vi "Attitude_ODE.vi"() -> ()   [LabVIEW 2018]
uses:
  <vilib>/Analysis/coordinate.llb/Euler Rotation Order.ctl
  <vilib>/imath/engines/lvmath2/RunTimeEngine/IndexRead/NIMS M(S,S).vi
  <instcachedir>/0/NIMS M(S,S)_AC51E74150A542F7991B9634C66F3096.lvgen/NIMS M(S,S)_AC51E74150A542F7991B9634C66F3096_002.vi
  <vilib>/imathl/engines/lvmath/Functions/Error Handling/Create Error.vi
  <vilib>/imath/engines/lvmath2/RunTimeEngine/IndexRead/NIMS V(S).vi
  <instcachedir>/0/NIMS V(S)_0488751826AF41519A22953C041130DC.lvgen/NIMS V(S)_0488751826AF41519A22953C041130DC_002.vi
  <vilib>/imath/engines/lvmath2/RunTimeEngine/ErrorHandling/NIMS_Create Error From Enums.vi
  <vilib>/imath/engines/lvmath2/RunTimeEngine/ArithmeticOperatorToken/NIMS_ArithmeticOperator_multmx-internal.vi
  <instcachedir>/0/NIMS_ArithmeticOperator_multmx-internal_16A6E1DA326644AB974D30232E729C42.lvgen/NIMS_ArithmeticOperator_multmx-internal_16A6E1DA326644AB974D30232E729C42_011.vi
  <instcachedir>/0/NIMS M(S,S)_AC51E74150A542F7991B9634C66F3096.lvgen/NIMS M(S,S)_AC51E74150A542F7991B9634C66F3096_000.vi
  <vilib>/imath/engines/lvmath2/RunTimeEngine/NodeEndStatement/NIMS_NodeEndStatement_Output.vi
  <instcachedir>/0/NIMS_NodeEndStatement_Output_53EC0D466D134D7ABD903AC30B43404B.lvgen/NIMS_NodeEndStatement_Output_53EC0D466D134D7ABD903AC30B43404B_005.vi
  <instcachedir>/0/NIMS_NodeEndStatement_Output_53EC0D466D134D7ABD903AC30B43404B.lvgen/NIMS_NodeEndStatement_Output_53EC0D466D134D7ABD903AC30B43404B_011.vi
  <vilib>/imath/engines/lvmath2/RunTimeEngine/ErrorHandling/NIMS_Finalize Error.vi
  <instcachedir>/0/NIMS_NodeEndStatement_Output_53EC0D466D134D7ABD903AC30B43404B.lvgen/NIMS_NodeEndStatement_Output_53EC0D466D134D7ABD903AC30B43404B_002.vi
  <vilib>/gmath/NI_Gmath.lvlib
  <vilib>/Analysis/NI_AALPro.lvlib
panel:
  out "Euler Angles":cluster{"phi":dbl, "theta":dbl, "psi":dbl}
  in  "stop":bool
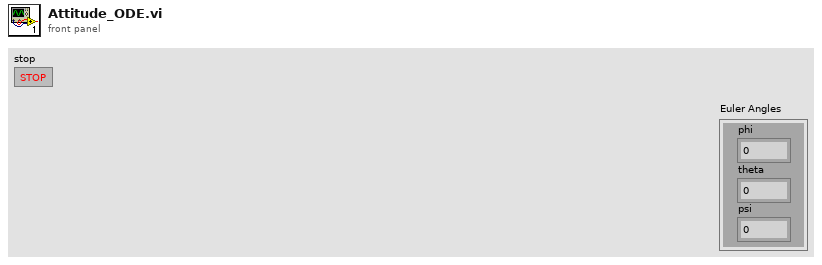
[diagram p1: front panel]
types:
  T1 = typedef "NI_AALPro.lvlib/Euler Rotation Order.ctl" = u16
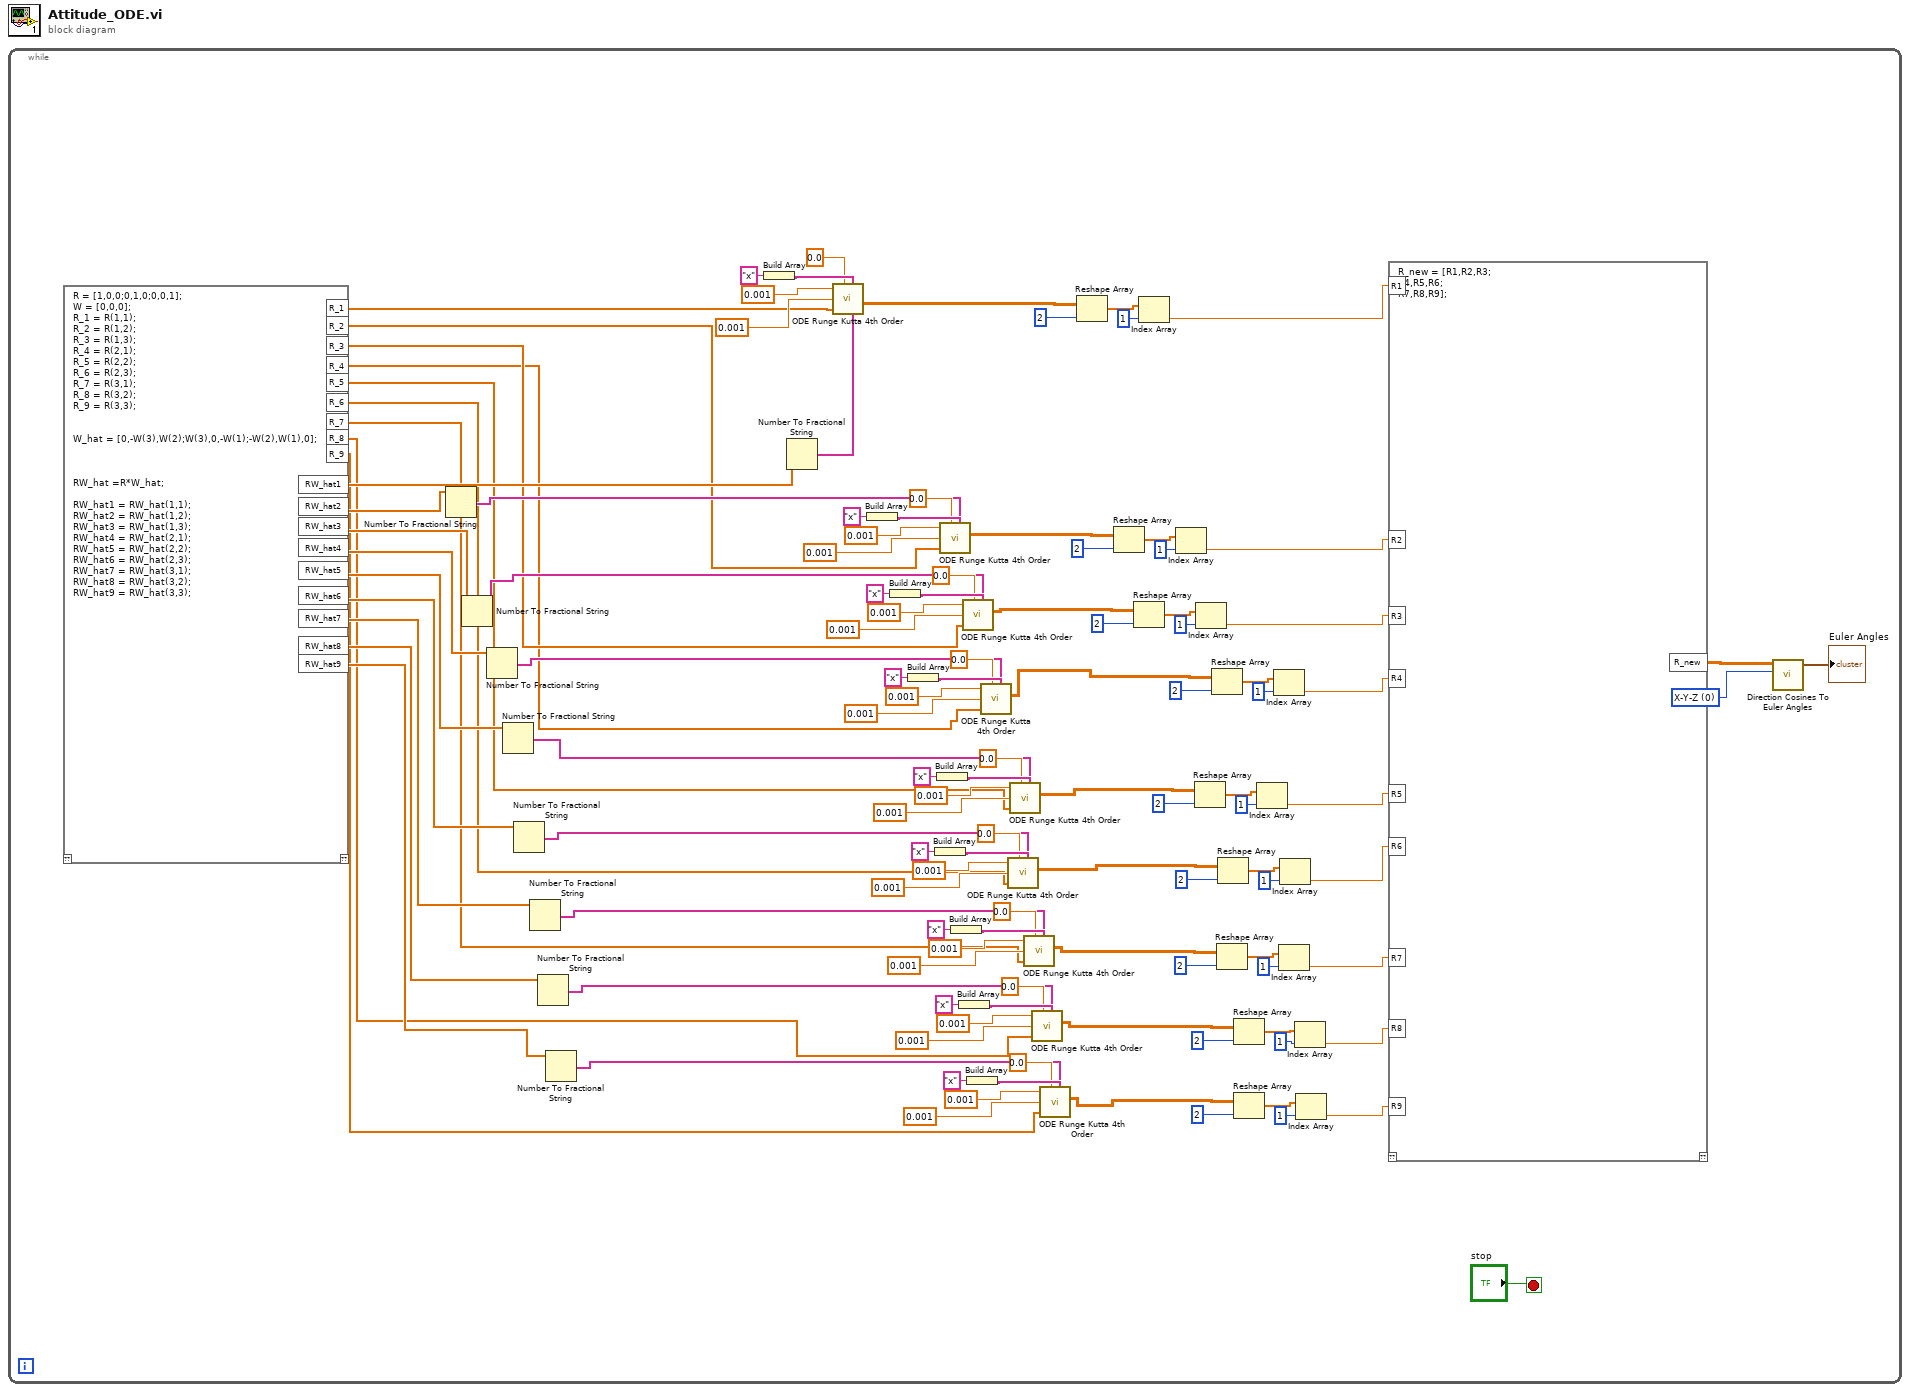
[diagram p0: block diagram]
diagram:
  n1 = while {
    stop <- "stop" stop-if-true
    w2 = T1 0 items=["X-Y-Z", "X-Z-Y", "Y-X-Z", "Y-Z-X", "Z-X-Y", "Z-Y-X", "X-Y-X", "X-Z-X", "Y-X-Y", "Y-Z-Y", "Z-X-Z", "Z-Y-Z"] ("rotation order")
    n2 = mathscript code="R = [1,0,0;0,1,0;0,0,1];\nW = [0,0,0];\nR_1 = R(1,1);\nR_2 = R(1,2);\nR_3 = R(1,3);\nR_4 = R(2,1);\nR_5 = R(2,2);\nR_6 = R(2,3);\nR_7 = R(3,1);\nR_8 = R(3,2);\nR_9 = R(3,3);\n\n\nW_hat = [0,-W(3),W(2);W(3),0,-W(1);-W(2),W(1),0];\n\n\n\nRW_hat =R*W_hat;\n\nRW_hat1 = RW_hat(1,1);\nRW_hat2 = RW_hat(1,2);\nRW_hat3 = RW_hat(1,3);\nRW_hat4 = RW_hat(2,1);\nRW_hat5 = RW_hat(2,2);\nRW_hat6 = RW_hat(2,3);\nRW_hat7 = RW_hat(3,1);\nRW_hat8 = RW_hat(3,2);\nRW_hat9 = RW_hat(3,3);"() -> ("RW_hat1"=w114:dbl[], "R_1"=w113:dbl[], "RW_hat2"=w107:dbl[], "RW_hat3"=w99:dbl[], "RW_hat4"=w92:dbl[], "RW_hat5"=w85:dbl[], "RW_hat6"=w78:dbl[], "RW_hat7"=w71:dbl[], "RW_hat8"=w64:dbl[], "RW_hat9"=w57:dbl[], "R_2"=w56:dbl[], "R_3"=w55:dbl[], "R_4"=w54:dbl[], "R_5"=w53:dbl[], "R_6"=w52:dbl[], "R_7"=w51:sgl[], "R_8"=w50:dbl[], "R_9"=w49:dbl[])  [unwired: 1 in, 1 out]
    n3 = Number To Fractional String(number=w107) -> (F-format string=w106:string[])  [unwired: 3 in]
    n4 = Number To Fractional String(number=w99) -> (F-format string=w100:string[])  [unwired: 3 in]
    n5 = Number To Fractional String(number=w92) -> (F-format string=w93:string[])  [unwired: 3 in]
    n6 = Number To Fractional String(number=w85) -> (F-format string=w86:string[])  [unwired: 3 in]
    n7 = Number To Fractional String(number=w78) -> (F-format string=w79:string[])  [unwired: 3 in]
    n8 = Number To Fractional String(number=w71) -> (F-format string=w72:string[])  [unwired: 3 in]
    n9 = Number To Fractional String(number=w64) -> (F-format string=w65:string[])  [unwired: 3 in]
    n10 = Number To Fractional String(number=w57) -> (F-format string=w58:string[])  [unwired: 3 in]
    n11 = Build Array("x") -> (w120:string[])
    n12 = Number To Fractional String(number=w114) -> (F-format string=w115:string[])  [unwired: 3 in]
    n13 = call <vilib>:"ODE Runge Kutta 4th Order.vi"("time end"=0.001, "time start"=0.0, "h (step rate)"=0.001, "X0"=w113, "X (name of variables)"=w120, "F(X,t) (right sides of the ODE\nas functions of X and t)"=w115) -> ("X Values (solution)"=w41:dbl[][])  [unwired: 1 in, 3 out]
    n14 = Build Array("x") -> (w111:string[])
    n15 = Build Array("x") -> (w104:string[])
    n16 = Build Array("x") -> (w97:string[])
    n17 = Build Array("x") -> (w83:string[])
    n18 = Build Array("x") -> (w90:string[])
    n19 = call <vilib>:"ODE Runge Kutta 4th Order.vi"("time end"=0.001, "time start"=0.0, "h (step rate)"=0.001, "X0"=w56, "X (name of variables)"=w111, "F(X,t) (right sides of the ODE\nas functions of X and t)"=w106) -> ("X Values (solution)"=w37:dbl[][])  [unwired: 1 in, 3 out]
    n20 = Build Array("x") -> (w76:string[])
    n21 = Build Array("x") -> (w69:string[])
    n22 = call <vilib>:"ODE Runge Kutta 4th Order.vi"("time end"=0.001, "time start"=0.0, "h (step rate)"=0.001, "X0"=w55, "X (name of variables)"=w104, "F(X,t) (right sides of the ODE\nas functions of X and t)"=w100) -> ("X Values (solution)"=w33:dbl[][])  [unwired: 1 in, 3 out]
    n23 = Build Array("x") -> (w62:string[])
    n24 = call <vilib>:"ODE Runge Kutta 4th Order.vi"("time end"=0.001, "time start"=0.0, "h (step rate)"=0.001, "X0"=w54, "X (name of variables)"=w97, "F(X,t) (right sides of the ODE\nas functions of X and t)"=w93) -> ("X Values (solution)"=w48:dbl[][])  [unwired: 1 in, 3 out]
    n25 = call <vilib>:"ODE Runge Kutta 4th Order.vi"("time end"=0.001, "time start"=0.0, "h (step rate)"=0.001, "X0"=w52, "X (name of variables)"=w83, "F(X,t) (right sides of the ODE\nas functions of X and t)"=w79) -> ("X Values (solution)"=w25:dbl[][])  [unwired: 1 in, 3 out]
    n26 = call <vilib>:"ODE Runge Kutta 4th Order.vi"("time end"=0.001, "time start"=0.0, "h (step rate)"=0.001, "X0"=w53, "X (name of variables)"=w90, "F(X,t) (right sides of the ODE\nas functions of X and t)"=w86) -> ("X Values (solution)"=w29:dbl[][])  [unwired: 1 in, 3 out]
    n27 = call <vilib>:"ODE Runge Kutta 4th Order.vi"("time end"=0.001, "time start"=0.0, "h (step rate)"=0.001, "X0"=w51, "X (name of variables)"=w76, "F(X,t) (right sides of the ODE\nas functions of X and t)"=w72) -> ("X Values (solution)"=w21:dbl[][])  [unwired: 1 in, 3 out]
    n28 = call <vilib>:"ODE Runge Kutta 4th Order.vi"("time end"=0.001, "time start"=0.0, "h (step rate)"=0.001, "X0"=w50, "X (name of variables)"=w69, "F(X,t) (right sides of the ODE\nas functions of X and t)"=w65) -> ("X Values (solution)"=w17:dbl[][])  [unwired: 1 in, 3 out]
    n29 = call <vilib>:"ODE Runge Kutta 4th Order.vi"("time end"=0.001, "time start"=0.0, "h (step rate)"=0.001, "X0"=w49, "X (name of variables)"=w62, "F(X,t) (right sides of the ODE\nas functions of X and t)"=w58) -> ("X Values (solution)"=w13:dbl[][])  [unwired: 1 in, 3 out]
    n30 = Reshape Array(w41, 2 ("dimension size")) -> (w43:dbl[])
    n31 = Reshape Array(w37, 2 ("dimension size")) -> (w39:dbl[])
    n32 = Reshape Array(w33, 2 ("dimension size")) -> (w35:dbl[])
    n33 = Index Array(array=w43, index=1) -> (element=w12:dbl)
    n34 = Index Array(array=w39, index=1) -> (element=w11:dbl)
    n35 = Reshape Array(w29, 2 ("dimension size")) -> (w31:dbl[])
    n36 = Index Array(array=w35, index=1) -> (element=w10:dbl)
    n37 = Reshape Array(w48, 2 ("dimension size")) -> (w46:dbl[])
    n38 = Reshape Array(w21, 2 ("dimension size")) -> (w23:dbl[])
    n39 = Reshape Array(w25, 2 ("dimension size")) -> (w27:dbl[])
    n40 = Reshape Array(w17, 2 ("dimension size")) -> (w19:dbl[])
    n41 = Reshape Array(w13, 2 ("dimension size")) -> (w15:dbl[])
    n42 = Index Array(array=w31, index=1) -> (element=w8:dbl)
    n43 = Index Array(array=w46, index=1) -> (element=w9:dbl)
    n44 = Index Array(array=w23, index=1) -> (element=w6:dbl)
    n45 = Index Array(array=w27, index=1) -> (element=w7:dbl)
    n46 = Index Array(array=w19, index=1) -> (element=w5:dbl)
    n47 = Index Array(array=w15, index=1) -> (element=w4:dbl)
    n48 = mathscript code="R_new = [R1,R2,R3;\nR4,R5,R6;\nR7,R8,R9];"("R1"=w12, "R2"=w11, "R3"=w10, "R4"=w9, "R5"=w8, "R6"=w7, "R7"=w6, "R8"=w5, "R9"=w4) -> ("R_new"=w3:dbl[][])  [unwired: 1 in, 1 out]
    n49 = call <vilib>:"Direction Cosines To Euler Angles.vi"("rotation order"=w2, "Direction Cosines"=w3) -> ("Euler Angles"=→"Euler Angles":cluster{"phi":dbl, "theta":dbl, "psi":dbl})  [unwired: 8 in, 1 out]
  }
